vi "Read PL txt File 2.vi"(1 "Path":path) -> (0 "XY Graph":cluster{"all rows":dbl[], "all rows":dbl[]}(graph))   [LabVIEW 2011]
uses:
  <vilib>/Utility/file.llb/Read From Spreadsheet File (DBL).vi
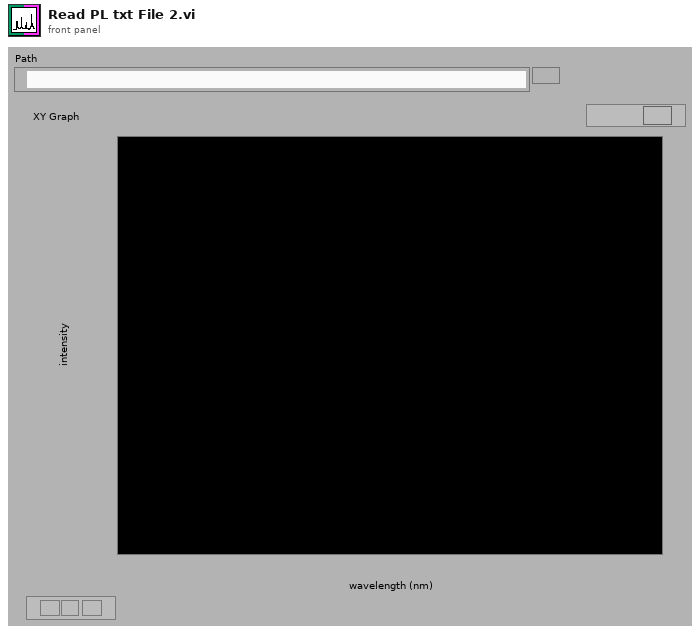
[diagram p1: front panel]
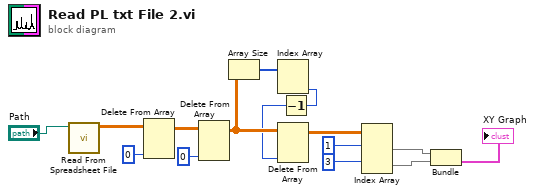
[diagram p0: block diagram]
diagram:
  n1 = call-poly <vilib>:"Read From Spreadsheet File.vi"("file path (dialog if empty)"="Path") -> ("all rows"=w10:dbl[][])  [unwired: 3 in, 7 out]
  n2 = Delete From Array(array=w10, index (col)=0 ("disabled index (col)")) -> (array with subset deleted=w13:dbl[][])  [unwired: 2 in, 1 out]
  n3 = Delete From Array(array=w13, index (col)=0 ("disabled index (col)")) -> (array with subset deleted=w4:dbl[][])  [unwired: 2 in, 1 out]
  n4 = Array Size(array=w4) -> (size(s)=w3:i32[])
  n5 = Index Array(array=w3) -> (element #2=w2:i32)  [unwired: 2 in, 1 out]
  n6 = Decrement(x=w2) -> (x-1=w1:i32)
  n7 = Delete From Array(array=w4, index (col)=w1) -> (array with subset deleted=w14:dbl[][])  [unwired: 2 in, 1 out]
  n8 = Index Array(array=w14, index (row) #1=1 ("index (row)"), index (row) #2=3 ("index (row)")) -> (element #1=w9:dbl[], element #2=w8:dbl[])  [unwired: 2 in]
  n9 = Bundle("all rows"=w9, "all rows"=w8) -> (→"XY Graph":cluster{"all rows":dbl[], "all rows":dbl[]})  [unwired: 1 out]
